vi "PowerSensor_ReadPower.vi"(8 "error in":errorcluster) -> (0 "error out":errorcluster, 3 "Response":string)   [LabVIEW 2023, in "Anritsu.lvlib"]
uses:
  Anritsu.lvlib
panel:
  in  "VISA in":refnum<visa-resource-name>="USB0::0x0B5B::0xFF82::1809045::RAW"
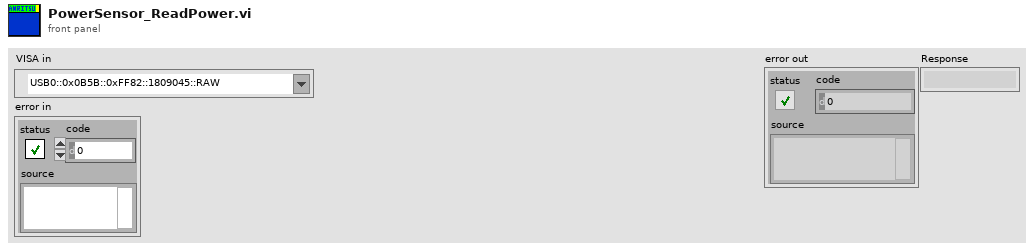
[diagram p1: front panel]
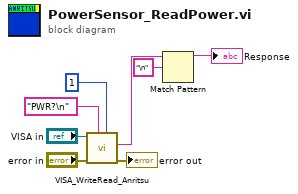
[diagram p0: block diagram]
diagram:
  n1 = call "VISA_WriteRead_Anritsu.vi"("waiting(ms)"=u32 1, "VISA_CMD"="PWR?\n", "error in"="error in", "VISA in"="VISA in") -> ("error out"=→"error out":errorcluster, "Response"=w3:string)  [unwired: 5 in, 1 out]
  n2 = Match Pattern(string=w3, regular expression="\n") -> (before substring=→"Response":string)  [unwired: 1 in, 3 out]
